vi "Generate Plot.vi"() -> (0 "Lower":cluster{"x":dbl[], "yl":dbl[]}, 1 "Upper":cluster{"x":dbl[], "yu":dbl[]})   [LabVIEW 2014]
uses:
  Labby Bird/Labby Bird/Labby bird-Support.llb/Global-1.vi
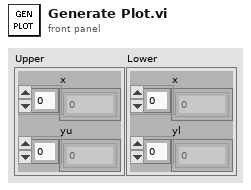
[diagram p1: front panel]
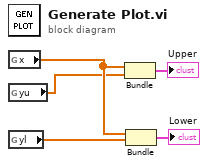
[diagram p0: block diagram]
diagram:
  n1 = global read "Global-1.vi" "x"() -> (w5:dbl[])
  n2 = global read "Global-1.vi" "yu"() -> (w4:dbl[])
  n3 = global read "Global-1.vi" "yl"() -> (w3:dbl[])
  n4 = Bundle("x"=w5, "yu"=w4) -> (→"Upper":cluster{"x":dbl[], "yu":dbl[]})  [unwired: 1 in]
  n5 = Bundle("x"=w5, "yl"=w3) -> (→"Lower":cluster{"x":dbl[], "yl":dbl[]})  [unwired: 1 in]
